vi "User Defined Type Class Server.vi"() -> ()   [LabVIEW 2020]
uses:
  My Custom Type/My Custom Type.lvclass
  source/Server/Server/Server.lvclass
  source/Server/Server/Fetch - User Defined.vi
  source/Server/Server/Add PV - Any Class.vi
  source/Server/Server/Post - Any Class.vi
  source/PV Data/EPICS Time Stamp.ctl
  source/PV Data/PV Data.lvlib
  Custom Structure.ctl
panel:
  in  "Cluster":T1
  in  "PV name":string="DEV:NDLT2043:STRUCT"
  in  "stop":bool
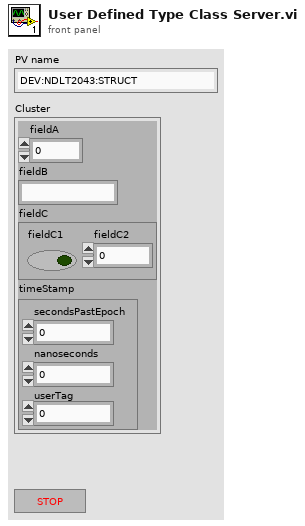
[diagram p1: front panel]
types:
  T1 = typedef "Custom Structure.ctl" = cluster{"fieldA":i32, "fieldB":string, "fieldC":cluster{"fieldC1":bool, "fieldC2":dbl}, "timeStamp":T2}
  T2 = typedef "PV Access.lvlib/PV Data.lvlib/EPICS Time Stamp.ctl" = cluster{"secondsPastEpoch":i64, "nanoseconds":i32, "userTag":i32}
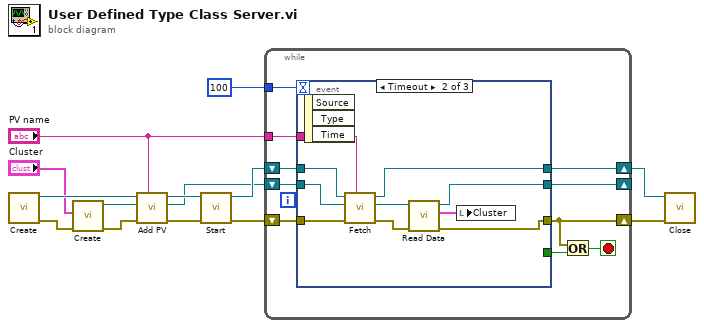
[diagram p0: block diagram]
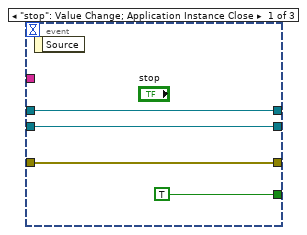
[diagram p2: hidden frame]
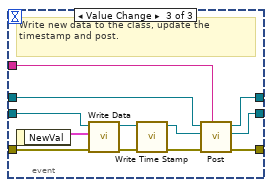
[diagram p3: hidden frame]
diagram:
  n1 = call "Create.vi"() -> ("error out"=w2:errorcluster, "Server out"=w11:refnum<class "Server.lvclass">)  [unwired: 10 in]
  n2 = call "Create.vi"("error in (no error)"=w2, "data"="Cluster") -> ("error out"=w3:errorcluster, "My Custom Type out"=w4:refnum<class "My Custom Type.lvclass">)  [unwired: 8 in]
  n3 = call-poly "Add PV.vi"("PV name"="PV name", "error in (no error)"=w3, "initial value"=w4, "Server in"=w11) -> ("error out"=w9:errorcluster, "value out"=w5:refnum<class "My Custom Type.lvclass">, "Server out"=w8:refnum<class "Server.lvclass">)  [unwired: 5 in]
  n4 = call-dynamic "Start.vi"("error in (no error)"=w9, "Server in"=w8) -> ("error out"=w6:errorcluster, "Server out"=w7:refnum<class "Server.lvclass">)  [unwired: 8 in]
  n5 = while {
    tunnel: "PV name" -> [w23]
    shift-right: [w21] -> w12
    shift-left: w7 -> [w22]
    shift-right: [w18] -> w13
    shift-left: w6 -> [w24]
    tunnel: 100 ("Numeric") -> [w17]
    shift-right: [w15] -> _
    shift-left: w5 -> [w16]
    stop <- w19 stop-if-true
    n6 = event shown="[1] Timeout" {
      selector: _ -> [_ _ _]
      dyn-events: _ -> [_ _ _]
      timeout: w17 -> [_ _ _]
      tunnel: w24 -> [w27 w38 w40]
      tunnel: w23 -> [_ w35 w49]
      tunnel: w22 -> [w26 w37 w44]
      tunnel: [w27 w31 w50] -> w18
      tunnel: [w26 w36 w48] -> w21
      tunnel: [TRUE _ _] -> w20
      tunnel: w16 -> [w25 w34 w42]
      tunnel: [w25 w29 w39] -> w15
      event "stop": Value Change; Application Instance Close {
        n7 = event-data() -> ()  [unwired: 1 in, 1 out]
      }
      event Timeout {
        n8 = event-data() -> ()  [unwired: 1 in, 3 out]
        n9 = call-poly "Fetch.vi"("PV name"=w35, "error in"=w38, "default value"=w34, "Server in"=w37) -> ("error out"=w33:errorcluster, "value"=w32:refnum<class "My Custom Type.lvclass">, "Server out"=w36:refnum<class "Server.lvclass">)  [unwired: 4 in, 1 out]
        n10 = call-dynamic "Read Data.vi"("error in (no error)"=w33, "My Custom Type in"=w32) -> ("error out"=w31:errorcluster, "data"=w30:T1, "My Custom Type out"=w29:refnum<class "My Custom Type.lvclass">)  [unwired: 7 in]
        n11 = local write "Cluster"(w30) -> ()
      }
      event Value Change {
        # "Write new data to the class, update the timestamp and post."
        n12 = event-data() -> ("NewVal"=w47:T1)  [unwired: 1 in]
        n13 = call-dynamic "Write Data.vi"("error in (no error)"=w40, "data"=w47, "My Custom Type in"=w42) -> ("error out"=w41:errorcluster, "My Custom Type out"=w43:refnum<class "My Custom Type.lvclass">)  [unwired: 7 in]
        n14 = call-dynamic "Write Time Stamp.vi"("error in"=w41, "Has Timestamp in"=w43) -> ("error out"=w46:errorcluster, "Has Timestamp out"=w45:refnum<class "My Custom Type.lvclass">)  [unwired: 8 in]
        n15 = call-poly "Post.vi"("PV name"=w49, "error in (no error)"=w46, "value in"=w45, "Server in"=w44) -> ("error out"=w50:errorcluster, "value out"=w39:refnum<class "My Custom Type.lvclass">, "Server out"=w48:refnum<class "Server.lvclass">)  [unwired: 5 in]
      }
    }
    n16 = Or(x=w18, y=w20) -> (x .or. y?=w19:bool)
  }
  n17 = call-dynamic "Close.vi"("error in"=w13, "Server in"=w12) -> ()  [unwired: 9 in, 1 out]
